vi "Set_Registers.vi"(2 "error in (no error)":errorcluster, 3 "Registers":T1 {"Reg1" format="0x%08x"; "Reg2" format="0x%08x"; "Reg3" format="0x%08x"; "Reg4" format="0x%08x"; "Reg5" format="0x%08x"; "Reg0" format="0x%08x"; "Reg6" format="0x%08x"}, 4 "VISA in":refnum<visa-resource-name>) -> (0 "error out":errorcluster, 1 "VISA out":refnum<visa-resource-name>)   [LabVIEW 2017, in "GP22_TDC_Arduinoed.lvlib"]
doc: "Set the GP22's internal registers to the given values. \n/* NOT IMPLEMENTED YET - If an input value of \"-1\" is given, the subVI will use ACAM's default settings for that register instead. */"
uses:
  GP22_TDC_Arduinoed.lvlib
  Registers.ctl
panel:
  out "Config string":string
  out "read buffer":string
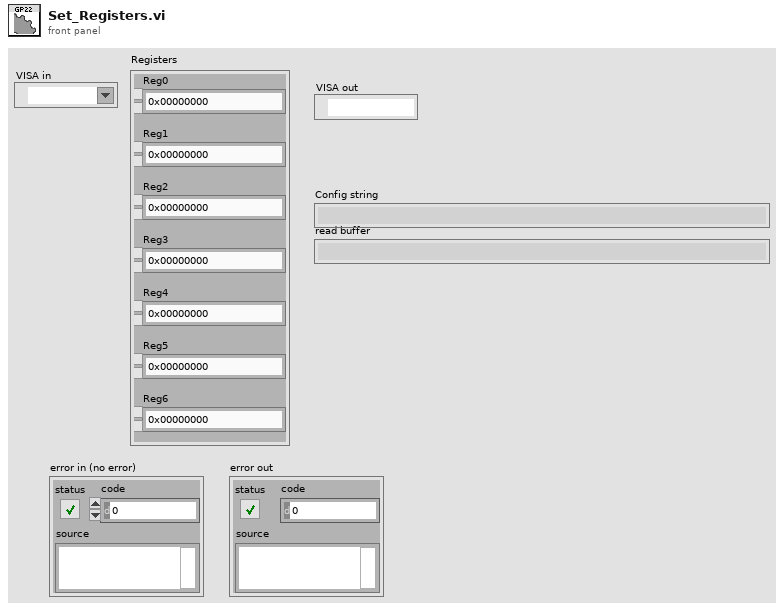
[diagram p1: front panel]
types:
  T1 = typedef "Registers.ctl" = cluster{"Reg0":u32, "Reg1":u32, "Reg2":u32, "Reg3":u32, "Reg4":u32, "Reg5":u32, "Reg6":u32}
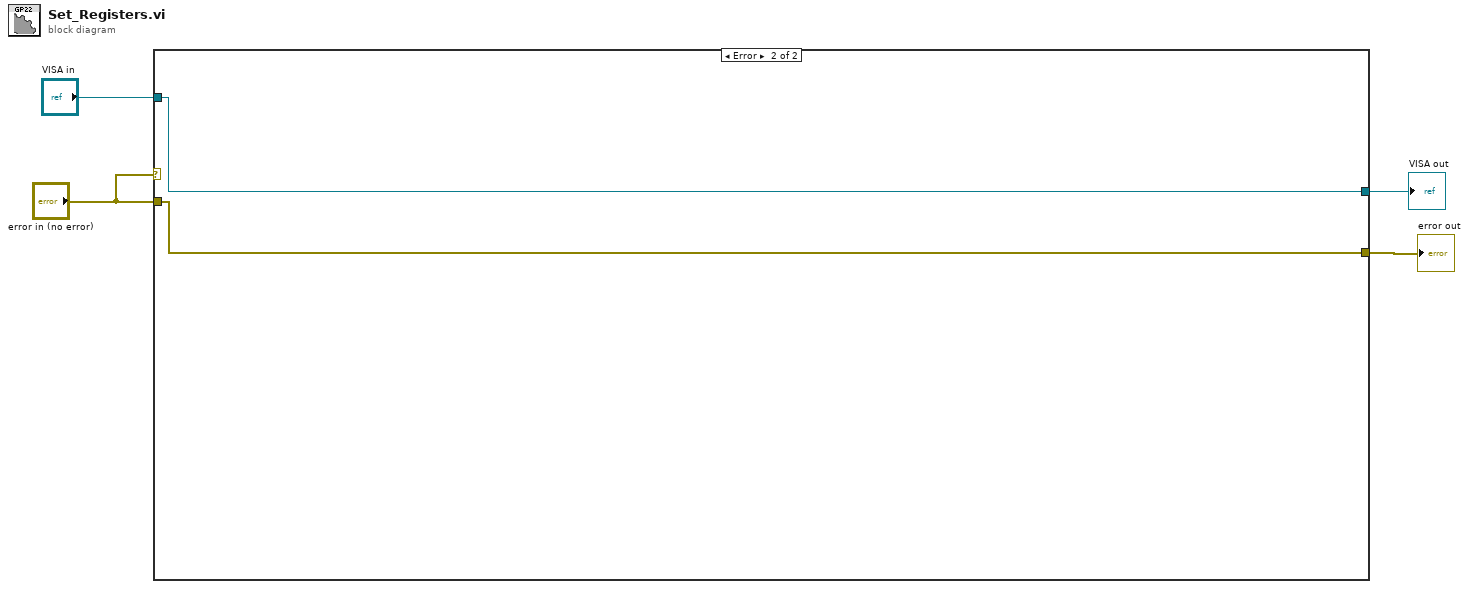
[diagram p0: block diagram]
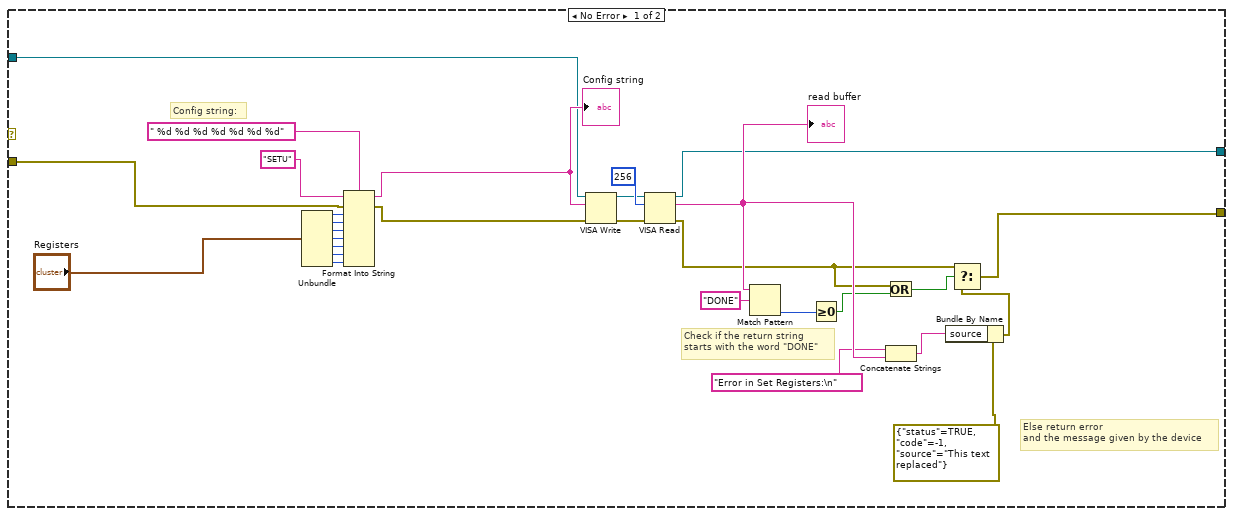
[diagram p2: hidden frame]
diagram:
  n1 = case shown="Error" "error in (no error)" {
    tunnel: [w31 w35] -> w4
    tunnel: "error in (no error)" -> [w24 w35]
    tunnel: [w6 w34] -> w2
    tunnel: "VISA in" -> [w5 w34]
    frame No Error {
      # "Config string:"
      # "Else return error\nand the message given by the device"
      # "Check if the return string\nstarts with the word \"DONE\""
      n2 = Unbundle("Registers") -> ("Reg0"=w19:u32, "Reg1"=w18:u32, "Reg2"=w17:u32, "Reg3"=w16:u32, "Reg4"=w15:u32, "Reg5"=w14:u32, "Reg6"=w13:u32)
      n3 = Format Into String(format string=" %d %d %d %d %d %d %d", initial string="SETU", error in=w24, w19, w18, w17, w16, w15, w14, w13) -> (resulting string=w26:string, error out=w25:errorcluster)
      "Config string" <- w26
      n4 = VISA Write(VISA resource name=w5, write buffer=w26, error in (no error)=w25) -> (VISA resource name out=w21:refnum<visa-resource-name>, error out=w27:errorcluster)  [unwired: 1 out]
      n5 = VISA Read(VISA resource name=w21, byte count=u32 256, error in (no error)=w27) -> (VISA resource name out=w6:refnum<visa-resource-name>, read buffer=w12:string, error out=w8:errorcluster)  [unwired: 1 out]
      "read buffer" <- w12
      n6 = Match Pattern(string=w12, regular expression="DONE") -> (offset past match=w30:i32)  [unwired: 1 in, 3 out]
      n7 = Greater Or Equal To 0?(x=w30) -> (x >= 0?=w9:bool)
      n8 = Or(x=w8, y=w9) -> (x .or. y?=w7:bool)
      n9 = Concatenate Strings("Error in Set Registers:\n" ("string"), w12) -> (w11:string)
      n10 = Bundle By Name(cluster=errorcluster {"status"=TRUE, "code"=-1, "source"="This text replaced"} ("f"), "source"=w11) -> (w33:errorcluster)
      n11 = Select(t=w8, s=w7, f=w33) -> (s? t:f=w31:errorcluster)
    }
    frame Error {
    }
  }
  "error out" <- w4
  "VISA out" <- w2
